vi "Attach Bus Monitor.vi"(10 "BusMonitor":refnum<class "IBusMonitor.lvclass">, 11 "MonitoredMediator in":refnum<class "MonitoredMediator.lvclass">) -> (3 "MonitoredMediator out":refnum<class "MonitoredMediator.lvclass">)   [LabVIEW 2020, in "MonitoredMediator.lvlib" / "MonitoredMediator.lvclass"]
uses:
  <vilib>/gpm_packages/@cs/mva-core/Source/MonitoredMediator/MonitoredMediator/MonitoredMediator.lvclass
  C:/Program Files/National Instruments/LabVIEW 2020/vi.lib/gpm_packages/@cs/mva-core/Source/Mediator/Mediator/Mediator.lvclass
  <vilib>/gpm_packages/@cs/mva-core/Source/MonitoredMediator/IBusMonitor/IBusMonitor.lvclass
  <vilib>/gpm_packages/@cs/mva-core/Source/MonitoredMediator/MonitoredMediator/MonitoredMediator.lvclass/MonitoredMediator.ctl
  <vilib>/gpm_packages/@cs/mva-core/Source/Mediator/Mediator/Mediator.lvclass/Mediator.ctl
  <vilib>/gpm_packages/@cs/mva-core/Source/Mediator/TopicLookupTable/TopicLookupTable.lvclass/TopicLookupTable.ctl
  <vilib>/gpm_packages/@cs/mva-core/Source/Mediator/Topic Messages/Add Topic Subscriber Msg/Add Topic Subscriber Msg.lvclass/Add Topic Subscriber Msg.ctl
  <vilib>/ActorFramework/Message Enqueuer/Message Enqueuer.lvclass/Message Enqueuer.ctl
  <vilib>/ActorFramework/Message Enqueuer/Enqueue.vi
  <vilib>/gpm_packages/@cs/mva-core/Source/Mediator/Topic Messages/Add Topic Subscriber Msg/Add Topic Subscriber Msg.lvclass
  C:/Program Files/National Instruments/LabVIEW 2020/vi.lib/ActorFramework/Message/Message.lvclass
  <vilib>/ActorFramework/Message Priority Queue/Priority Enqueue.vi
  <vilib>/ActorFramework/Message Enqueuer/Message Enqueuer.lvclass
  <vilib>/gpm_packages/@cs/mva-core/Source/Mediator/Mediator/Mediator.lvclass
  <vilib>/gpm_packages/@cs/mva-core/Source/Mediator/TopicLookupTable/TopicLookupTable.lvclass
  <vilib>/gpm_packages/@cs/mva-core/Source/IMediator/ISubscriptionPolicy/ISubscriptionPolicy.lvclass
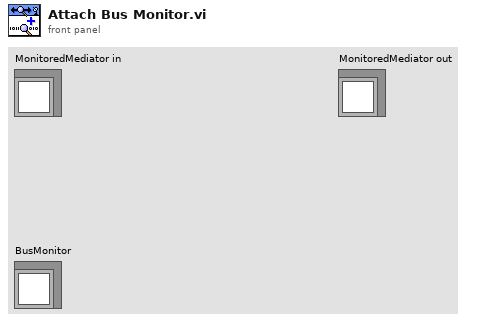
[diagram p1: front panel]
types:
  T1 = typedef "IMediator.lvlib/ISubscriptionPolicy.lvclass/ISubscriptionPolicy Reference.ctl" = refnum<data-value>
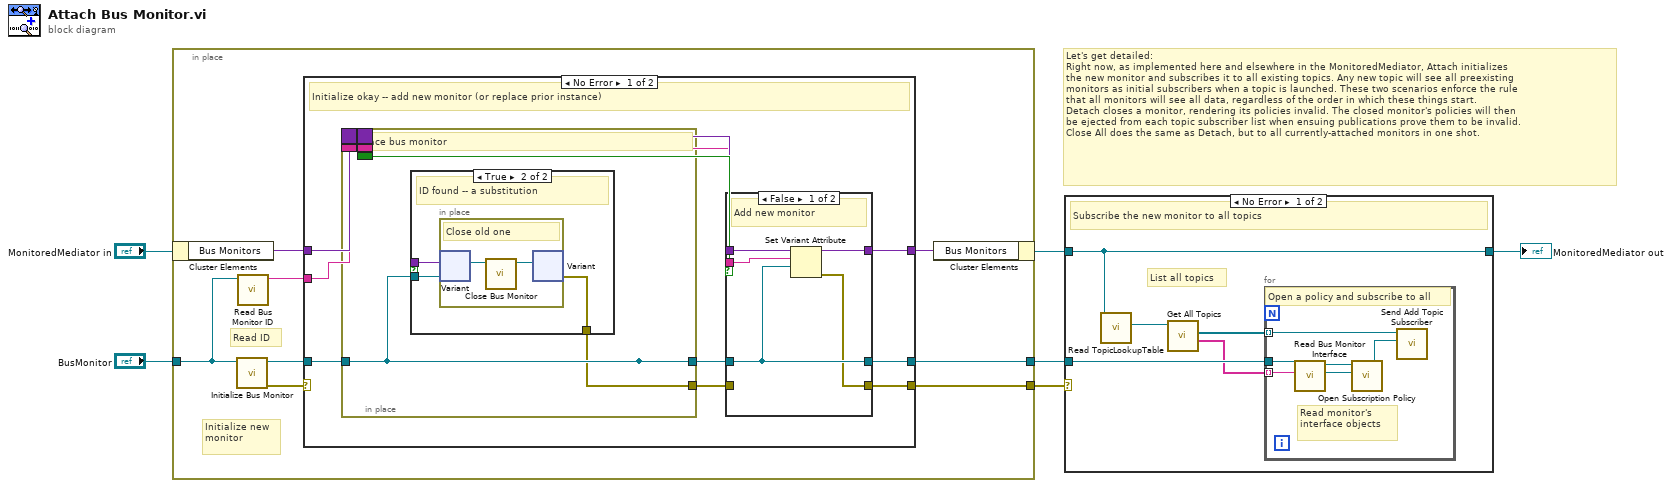
[diagram p0: block diagram]
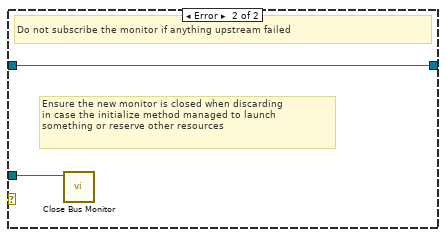
[diagram p5: hidden frame]
diagram:
  # "Let's get detailed:\nRight now, as implemented here and elsewhere in the MonitoredMediator, Attach initializes\nthe new monitor and subscribes it to all existing topics. Any new topic will see all preexisting\nmonitors as initial subscribers when a topic is launched. These two scenarios enforce the rule\nthat all monitors will see all data, regardless of the order in which these things start.\nDetach closes a monitor, rendering its policies invalid. The closed monitor's policies will then\nbe ejected from each topic subscriber list when ensuing publications prove them to be invalid.\nClose All does the same as Detach, but to all currently-attached monitors in one shot."
  n1 = in-place {
    in-place-border: "BusMonitor" -> [w8]
    in-place-border: [w10] -> w3
    in-place-border: [w7] -> w1
    # "Read ID"
    # "Initialize new\nmonitor"
    n2 = in-place-cluster #1("MonitoredMediator in") -> ("Bus Monitors"=w13:variant)
    n3 = call-dynamic "Initialize Bus Monitor.vi"("IBusMonitor In"=w8) -> ("error out"=w14:errorcluster, "IBusMonitor Out"=w12:refnum<class "IBusMonitor.lvclass">)  [unwired: 9 in]
    n4 = call-dynamic "Read Bus Monitor ID.vi"("IBusMonitor"=w8) -> ("Bus Monitor ID"=w9:string)  [unwired: 10 in]
    n5 = case shown="No Error" w14 {
      selector: w14 -> [_ w44]
      tunnel: w13 -> [w25 w45]
      tunnel: w12 -> [w24 w43]
      tunnel: [w19 w45] -> w11
      tunnel: [w18 w44] -> w10
      tunnel: w9 -> [w16 _]
      tunnel: [w15 w43] -> w7
      frame No Error {
        # "Initialize okay -- add new monitor (or replace prior instance)"
        n6 = in-place {
          border: w25 -> [_]
          border: w16 -> [_]
          border: [_] -> w22
          border: [_] -> w21
          border: [_] -> w23
          in-place-border: w24 -> [w35]
          in-place-border: [w35] -> w20
          in-place-border: [w34] -> w17
          # "Replace bus monitor"
          n7 = case shown="True" w36 {
            tunnel: w37 -> [_ w40]
            tunnel: w35 -> [_ w39]
            tunnel: [_ w38] -> w34
            frame False {
              # "Nothing to close"
              # "Old ID not found"
            }
            frame True {
              # "ID found -- a substitution"
              n8 = in-place {
                # "Close old one"
                n9 = in-place-variant #2(w40, w39) -> (w42:refnum<class "IBusMonitor.lvclass">)  [unwired: 1 out]
                n10 = call-dynamic "Close Bus Monitor.vi"("IBusMonitor In"=w42) -> ("IBusMonitor Out"=w41:refnum<class "IBusMonitor.lvclass">)  [unwired: 10 in]
                n11 = in-place-variant #2(w41) -> (w38:errorcluster)  [unwired: 1 out]
              }
            }
          }
        }
        n12 = case shown="False" w23 {
          tunnel: w22 -> [w30 w33]
          tunnel: w21 -> [w29 _]
          tunnel: w20 -> [w27 w31]
          tunnel: [w28 w33] -> w19
          tunnel: [w26 w32] -> w18
          tunnel: w17 -> [_ w32]
          tunnel: [w27 w31] -> w15
          frame False {
            # "Add new monitor"
            n13 = Set Variant Attribute(Variant=w30, name=w29, value=w27) -> (Variant out=w28:variant, error out=w26:errorcluster)  [unwired: 1 in, 1 out]
          }
          frame True {
            # "This was a substitution"
          }
        }
      }
      frame Error {
        # "Do not add new monitor if initialization fails"
      }
    }
    n14 = in-place-cluster #1("Bus Monitors"=w11) -> (w4:refnum<class "MonitoredMediator.lvclass">)
  }
  n15 = case shown="No Error" w3 {
    tunnel: w4 -> [w48 w58]
    tunnel: [w48 w58] -> w2
    tunnel: w1 -> [w47 w57]
    frame No Error {
      # "List all topics"
      # "Subscribe the new monitor to all topics"
      n16 = call <vilib>:"Read TopicLookupTable.vi"("Mediator in"=w48) -> ("TopicLookupTable"=w50:refnum<data-value>)  [unwired: 10 in]
      n17 = call <vilib>:"Get All Topics.vi"("TopicLookupTable"=w50) -> ("Topic Name"=w46:string[], "Topic Enqueuers"=w49:refnum<class "Message Enqueuer.lvclass">[])  [unwired: 7 in, 2 out]
      n18 = for {
        tunnel: w49 -> [w56] mode=indexing
        tunnel: w47 -> [w54]
        tunnel: w46 -> [w51] mode=indexing
        # "Read monitor's\ninterface objects"
        # "Open a policy and subscribe to all"
        n19 = call-dynamic "Read Bus Monitor Interface.vi"("Datum Name"=w51, "IBusMonitor"=w54) -> ("Valid Transport"=w53:refnum<class "ITransport.lvclass">, "SubscriptionPolicy Type"=w52:refnum<class "ISubscriptionPolicy.lvclass">)  [unwired: 8 in]
        n20 = call <vilib>:"Open Subscription Policy.vi"("Transport"=w53, "SubscriptionPolicy"=w52) -> ("Subscription Policy"=w55:T1)  [unwired: 8 in, 1 out]
        n21 = call <vilib>:"Send Add Topic Subscriber.vi"("Subscription Policy"=w55, "Message Enqueuer"=w56) -> ()  [unwired: 8 in, 2 out]
      }
    }
    frame Error {
      # "Ensure the new monitor is closed when discarding\nin case the initialize method managed to launch\nsomething or reserve other resources"
      # "Do not subscribe the monitor if anything upstream failed"
      n22 = call-dynamic "Close Bus Monitor.vi"("IBusMonitor In"=w57) -> ()  [unwired: 10 in, 1 out]
    }
  }
  "MonitoredMediator out" <- w2
